vi "Add1.vi"() -> ()   [LabVIEW 2019]
uses:
  Car Game/Supported.llb/Global-1.vi
panel:
  in  "Add":bool
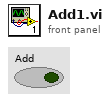
[diagram p1: front panel]
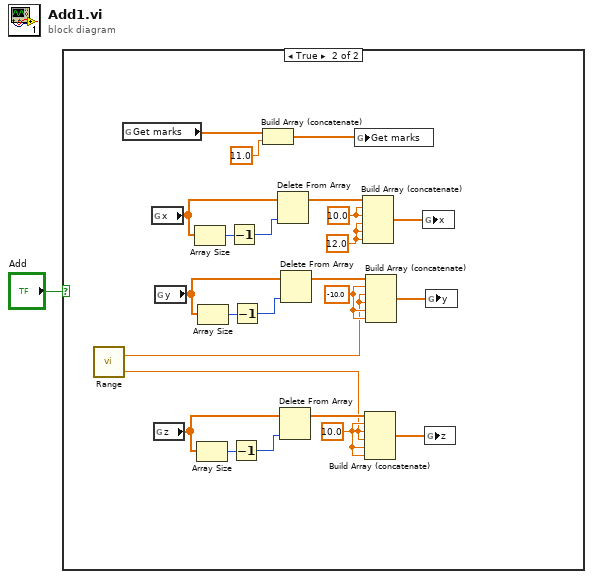
[diagram p0: block diagram]
diagram:
  n1 = case shown="True" "Add" {
    frame False {
    }
    frame True {
      w4 = 10.0
      w5 = -10.0
      w6 = 12.0
      w21 = 10.0
      n2 = call "Range.vi"() -> ("Lower"=w3:dbl, "Upper"=w2:dbl)  [unwired: 1 in]
      n3 = global read "Global-1.vi" "Get marks"() -> (w9:dbl[])
      n4 = global read "Global-1.vi" "x"() -> (w25:dbl[])
      n5 = global read "Global-1.vi" "z"() -> (w14:dbl[])
      n6 = global read "Global-1.vi" "y"() -> (w19:dbl[])
      n7 = Array Size(array=w25) -> (size(s)=w24:i32)
      n8 = Array Size(array=w14) -> (size(s)=w13:i32)
      n9 = Array Size(array=w19) -> (size(s)=w18:i32)
      n10 = Decrement(x=w24) -> (x-1=w23:i32)
      n11 = Decrement(x=w13) -> (x-1=w12:i32)
      n12 = Decrement(x=w18) -> (x-1=w17:i32)
      n13 = Build Array (concatenate)(w9, 11.0) -> (w8:dbl[])
      n14 = Delete From Array(array=w25, index=w23) -> (array with subset deleted=w22:dbl[])  [unwired: 1 in, 1 out]
      n15 = Delete From Array(array=w14, index=w12) -> (array with subset deleted=w11:dbl[])  [unwired: 1 in, 1 out]
      n16 = Delete From Array(array=w19, index=w17) -> (array with subset deleted=w16:dbl[])  [unwired: 1 in, 1 out]
      n17 = global write "Global-1.vi" "Get marks"(w8) -> ()
      n18 = Build Array (concatenate)(w22, w21, w21, w6, w6, w6) -> (w20:dbl[])
      n19 = Build Array (concatenate)(w11, w4, w2, w2, w4, w4) -> (w10:dbl[])
      n20 = Build Array (concatenate)(w16, w5, w3, w3, w5, w5) -> (w15:dbl[])
      n21 = global write "Global-1.vi" "x"(w20) -> ()
      n22 = global write "Global-1.vi" "z"(w10) -> ()
      n23 = global write "Global-1.vi" "y"(w15) -> ()
    }
  }
